vi "Message Handling Loop - UI.vi"(8 "error in":errorcluster, 9 "Message Queues in":T1, 10 "User Event Bundle":T2) -> (0 "error out":errorcluster)   [LabVIEW 2018]
uses:
  Type Defs/User Events.ctl
  Support/Message Queue/All Message Queues.ctl
  Support/Message Queue/Message Cluster.ctl
  Type Defs/UI Loop Data.ctl
  Type Defs/SR Cluster.ctl
  Type Defs/SR Status.ctl
  Type Defs/Filter Cluster.ctl
  Type Defs/Sorting Methods.ctl
  Support/Message Queue/Enqueue Message (Single).vi
  <vilib>/Utility/error.llb/Error Cluster From Error Code.vi
  <vilib>/ErrorRing/Error Ring.xnode
  Support/Message Queue/Message Queue.lvlib
  Support/User Events/User Events.lvlib
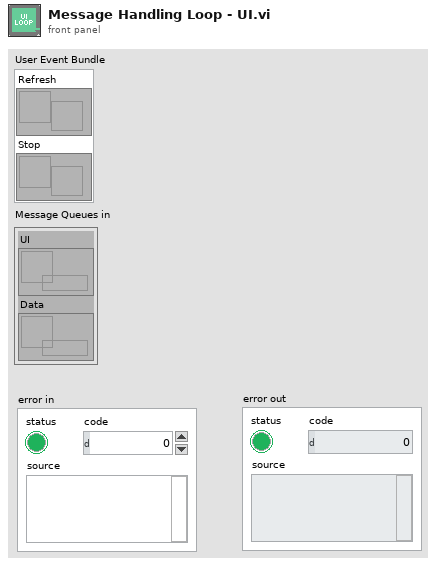
[diagram p1: front panel]
types:
  T1 = typedef "Message Queue.lvlib/All Message Queues.ctl" = cluster{"UI":refnum<queue>, "Data":refnum<queue>}
  T2 = typedef "User Events.ctl" = cluster{"Refresh":refnum<user-event>, "Stop":refnum<user-event>}
  T3 = typedef "UI Loop Data.ctl" = cluster{"SR Display List":T4[], "Filter Cluster":T6, "Exit":refnum<vi>, "Main VI":refnum<vi>, "Sorting":T7, "SR Display List":refnum<vi>, "Message":refnum<vi>, "UI":refnum<queue>, "Data":refnum<queue>}
  T4 = typedef "SR Cluster.ctl" = cluster{"Color":u32, "SR Number":i32, "SR Status":T5, "Name":string, "Summary":string, "Last Updated":timestamp, "SR Type":string, "Service Level":string, "Days Open":dbl, "Creation Date":timestamp}
  T5 = typedef "SR Status.ctl" = enum16{"Caller Abandoned", "Created in Error", "Expired", "Forum Resolved AE", "Forum Resolved Customer", "IN WORK", "IN WORK Collab with AES", "IN WORK Collab with PSE", "IN WORK Collab with SE", "IN WORK Customer Added Note", "IN WORK Escalation", "IN WORK Wait on Customer", "Open", "Potentially Resolved", "Presumed Resolved", "RMA Approved for Return", "Resolved", "Passed Off"}
  T6 = typedef "Filter Cluster.ctl" = cluster{"Show Resolved":bool, "Show Potentially Resolved":bool, "Show Passoffs":bool, "Show In Collab":bool}
  T7 = typedef "Sorting Methods.ctl" = enum16{"SR Status", "Most Recent", "SR Type", "SR Number"}
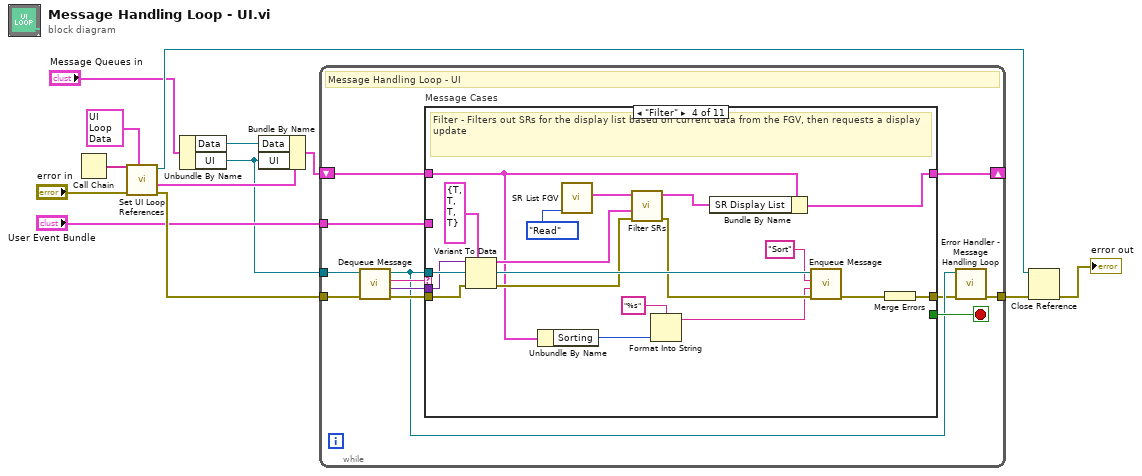
[diagram p0: block diagram]
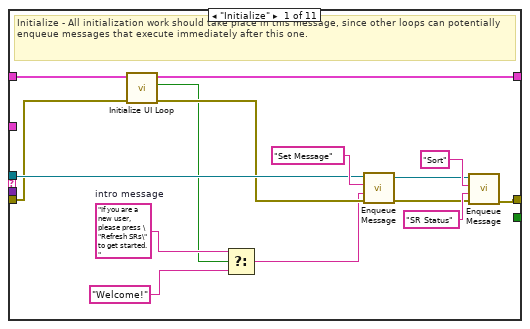
[diagram p2: hidden frame]
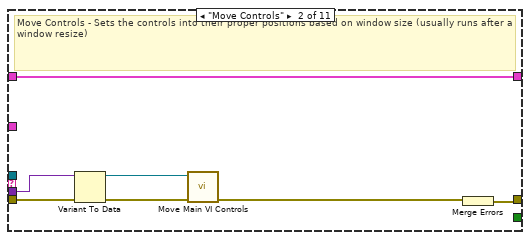
[diagram p3: hidden frame]
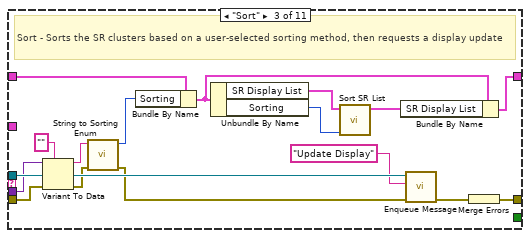
[diagram p4: hidden frame]
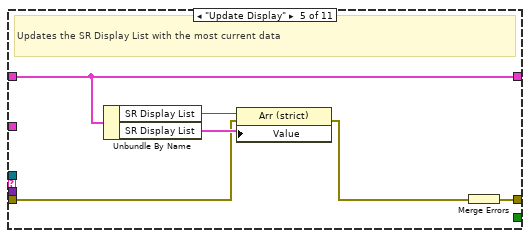
[diagram p5: hidden frame]
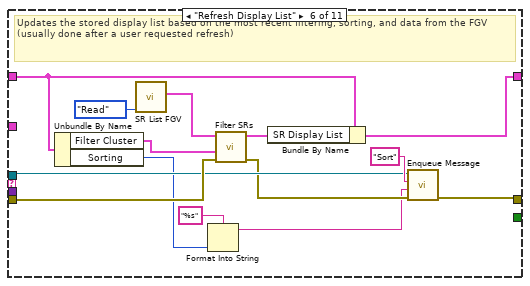
[diagram p6: hidden frame]
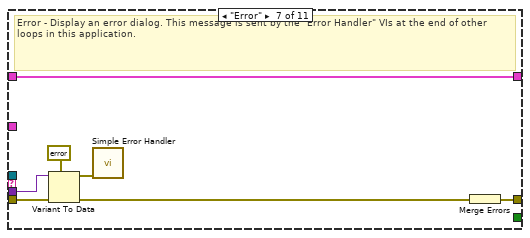
[diagram p7: hidden frame]
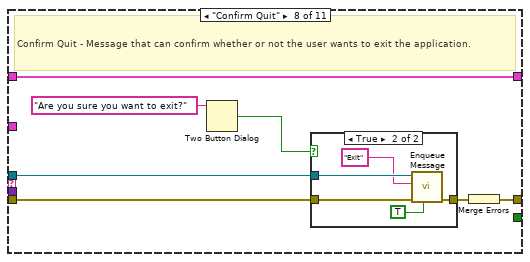
[diagram p8: hidden frame]
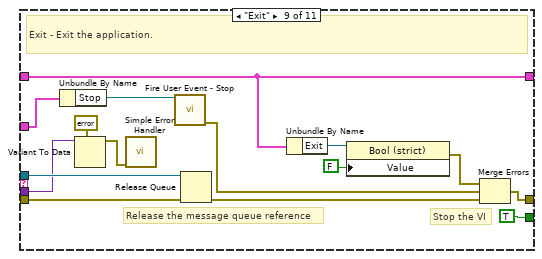
[diagram p10: hidden frame]
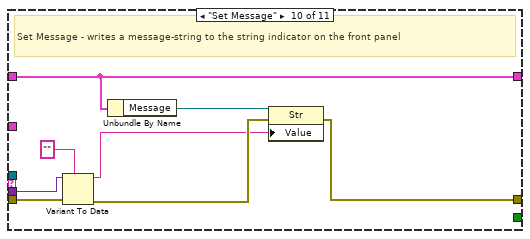
[diagram p11: hidden frame]
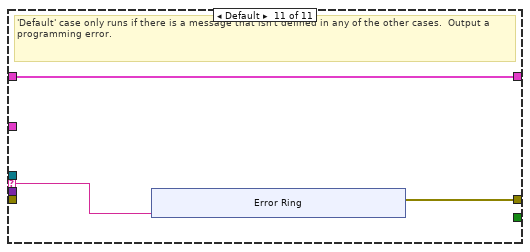
[diagram p12: hidden frame]
diagram:
  n1 = Call Chain() -> (call chain=w9:string[])
  n2 = call "Set UI Loop References.vi"("UI Data in"=T3 {"SR Display List"=[], "Filter Cluster"={"Show Resolved"=TRUE, "Show Potentially Resolved"=TRUE, "Show Passoffs"=TRUE, "Show In Collab"=TRUE}, "Exit"=refnum, "Main VI"=refnum, "Sorting"=enum."SR Status", "SR Display List"=refnum, "Message"=refnum, "UI"=refnum, "Data"=refnum}, "error in (no error)"="error in", "call chain"=w9) -> ("error out"=w13:errorcluster, "UI Data out"=w4:T3, "VI reference out"=w12:refnum<vi>)  [unwired: 6 in]
  n3 = Unbundle By Name("Message Queues in") -> ("Data"=w5:refnum<queue>, "UI"=w3:refnum<queue>)
  n4 = Bundle By Name(cluster=w4, "Data"=w5, "UI"=w3) -> (w1:T3)
  n5 = while {
    tunnel: w3 -> [w18]
    shift-right: [w24] -> _
    shift-left: w1 -> [w25]
    tunnel: w13 -> [w22]
    tunnel: [w16] -> w10
    tunnel: "User Event Bundle" -> [w14]
    stop <- w23 stop-if-true
    # "Message Handling Loop - UI"
    n6 = call "Dequeue Message.vi"("error in (no error)"=w22, "Message Queue"=w18) -> ("error out"=w21:errorcluster, "Message Data"=w19:variant, "Message"=w20:string, "dup Message Queue"=w17:refnum<queue>)  [unwired: 6 in]
    n7 = case "Message Cases" shown="\"Filter\"" w20 {
      selector: w20 -> [_ _ _ _ _ _ _ _ _ _ w146]
      tunnel: w17 -> [w34 _ w62 w80 _ w96 _ w112 w137 _ _]
      tunnel: w21 -> [w33 w46 w57 w71 w84 w98 w109 w116 w134 w143 _]
      tunnel: [w40 w42 w64 w82 w88 w94 w103 w114 w127 w139 w147] -> w15
      tunnel: w25 -> [w38 w47 w50 w68 w87 w93 w108 w115 w130 w145 w148]
      tunnel: [w39 w47 w59 w74 w87 w99 w108 w115 w130 w145 w148] -> w24
      tunnel: [_ _ _ _ _ _ _ _ TRUE _ _] -> w23
      tunnel: w19 -> [_ w44 w58 w72 _ _ w107 _ w131 w142 _]
      tunnel: w14 -> [_ _ _ _ _ _ _ _ w125 _ _]
      frame "Initialize" {
        w29 = "If you are a new user, please press \"Refresh SRs\" to get started."  # intro message
        # "Initialize - All initialization work should take place in this message, since other loops can potentially enqueue messages that execute immediately after this one."
        n8 = call "Initialize UI Loop.vi"("error in"=w33, "UI Data in"=w38) -> ("error out"=w32:errorcluster, "new user?"=w26:bool, "UI Data out 2"=w39:T3)  [unwired: 7 in]
        n9 = Select(t=w29, s=w26, f="Welcome!") -> (s? t:f=w27:string)
        n10 = call-poly "Enqueue Message.vi"("error in (no error)"=w32, "Message Data"=w27, "Message"="Set Message", "Message Queue"=w34) -> ("error out"=w31:errorcluster, "dup Message Queue"=w30:refnum<queue>)  [unwired: 6 in]
        n11 = call-poly "Enqueue Message.vi"("error in (no error)"=w31, "Message Data"="SR Status" ("Message"), "Message"="Sort", "Message Queue"=w30) -> ("error out"=w40:errorcluster)  [unwired: 6 in, 1 out]
      }
      frame "Move Controls" {
        # "Move Controls - Sets the controls into their proper positions based on window size (usually runs after a window resize)"
        n12 = Variant To Data(error in=w46, Variant=w44) -> (data=w45:refnum<vi>, error out=w43:errorcluster)  [unwired: 1 in]
        n13 = call "Move Main VI Controls.vi"("error in"=w43, "VIRef in"=w45) -> ("error out"=w41:errorcluster)  [unwired: 9 in]
        n14 = Merge Errors(w41) -> (w42:errorcluster)
      }
      frame "Sort" {
        # "Sort - Sorts the SR clusters based on a user-selected sorting method, then requests a display update"
        n15 = Variant To Data(error in=w57, type="", Variant=w58) -> (data=w56:string, error out=w54:errorcluster)
        n16 = call "String to Sorting Enum.vi"("error in"=w54, "string in"=w56) -> ("error out"=w53:errorcluster, "Sorting"=w49:T7)  [unwired: 8 in]
        n17 = Bundle By Name(cluster=w50, "Sorting"=w49) -> (w48:T3)
        n18 = Unbundle By Name(w48) -> ("SR Display List"=w60:T4[], "Sorting"=w51:T7)
        n19 = call "Sort SR List.vi"("Sorting"=w51, "list in"=w60) -> ("list out"=w52:T4[])  [unwired: 9 in]
        n20 = Bundle By Name(cluster=w48, "SR Display List"=w52) -> (w59:T3)
        n21 = call-poly "Enqueue Message.vi"("error in (no error)"=w53, "Message"="Update Display", "Message Queue"=w62) -> ("error out"=w63:errorcluster)  [unwired: 7 in, 1 out]
        n22 = Merge Errors(w63) -> (w64:errorcluster)
      }
      frame "Filter" {
        # "Filter - Filters out SRs for the display list based on current data from the FGV, then requests a display update"
        n23 = Variant To Data(error in=w71, type=T6 {"Show Resolved"=TRUE, "Show Potentially Resolved"=TRUE, "Show Passoffs"=TRUE, "Show In Collab"=TRUE} ("Filter Cluster"), Variant=w72) -> (data=w69:T6, error out=w70:errorcluster)
        n24 = Unbundle By Name(w68) -> ("Sorting"=w66:T7)
        n25 = call "SR List FGV.vi"("Operation"=enum16{"Initialize", "Write", "Read", "Clear"}."Read") -> ("list out"=w77:T4[])  [unwired: 9 in, 1 out]
        n26 = call "Filter SRs.vi"("error in"=w70, "Filter Cluster"=w69, "list in"=w77) -> ("error out"=w78:errorcluster, "list out"=w75:T4[])  [unwired: 7 in]
        n27 = Format Into String(format string="%s", w66) -> (resulting string=w65:string)  [unwired: 2 in, 1 out]
        n28 = Bundle By Name(cluster=w68, "SR Display List"=w75) -> (w74:T3)
        n29 = call-poly "Enqueue Message.vi"("error in (no error)"=w78, "Message Data"=w65, "Message"="Sort", "Message Queue"=w80) -> ("error out"=w81:errorcluster)  [unwired: 6 in, 1 out]
        n30 = Merge Errors(w81) -> (w82:errorcluster)
      }
      frame "Update Display" {
        # "Updates the SR Display List with the most current data"
        n31 = Unbundle By Name(w87) -> ("SR Display List"=w86:refnum<vi>, "SR Display List"=w85:T4[])
        n32 = property class="Arr (strict)"(reference=w86, error in=w84, "Value"=w85) -> (error out=w83:errorcluster)  [unwired: 1 out]
        n33 = Merge Errors(w83) -> (w88:errorcluster)
      }
      frame "Refresh Display List" {
        # "Updates the stored display list based on the most recent filtering, sorting, and data from the FGV (usually done after a user requested refresh)"
        n34 = Unbundle By Name(w93) -> ("Filter Cluster"=w90:T6, "Sorting"=w89:T7)
        n35 = call "SR List FGV.vi"("Operation"=enum16{"Initialize", "Write", "Read", "Clear"}."Read") -> ("list out"=w101:T4[])  [unwired: 9 in, 1 out]
        n36 = Format Into String(format string="%s", w89) -> (resulting string=w91:string)  [unwired: 2 in, 1 out]
        n37 = call "Filter SRs.vi"("error in"=w98, "Filter Cluster"=w90, "list in"=w101) -> ("error out"=w95:errorcluster, "list out"=w100:T4[])  [unwired: 7 in]
        n38 = Bundle By Name(cluster=w93, "SR Display List"=w100) -> (w99:T3)
        n39 = call-poly "Enqueue Message.vi"("error in (no error)"=w95, "Message Data"=w91, "Message"="Sort", "Message Queue"=w96) -> ("error out"=w94:errorcluster)  [unwired: 6 in, 1 out]
      }
      frame "Error" {
        # "Error - Display an error dialog. This message is sent by the \"Error Handler\" VIs at the end of other loops in this application."
        n40 = Variant To Data(error in=w109, type=errorcluster {"status"=FALSE, "code"=0, "source"=""} ("error constant"), Variant=w107) -> (data=w105:errorcluster, error out=w104:errorcluster)
        n41 = call <vilib>:"Simple Error Handler.vi"("error in (no error)"=w105) -> ()  [unwired: 4 in, 5 out]
        n42 = Merge Errors(w104) -> (w103:errorcluster)
      }
      frame "Confirm Quit" {
        # "Confirm Quit - Message that can confirm whether or not the user wants to exit the application."
        n43 = Two Button Dialog(message="Are you sure you want to exit?") -> (T button?=w110:bool)  [unwired: 2 in]
        n44 = case shown="True" w110 {
          tunnel: w116 -> [w117 w122]
          tunnel: [w117 w121] -> w113
          tunnel: w112 -> [_ w120]
          frame False {
          }
          frame True {
            n45 = call-poly "Enqueue Message.vi"("Priority Message? (F)"=TRUE, "error in (no error)"=w122, "Message"="Exit", "Message Queue"=w120) -> ("error out"=w121:errorcluster)  [unwired: 6 in, 1 out]
          }
        }
        n46 = Merge Errors(w113) -> (w114:errorcluster)
      }
      frame "Exit" {
        # "Stop the VI"
        # "Release the message queue reference"
        # "Exit - Exit the application."
        n47 = Unbundle By Name(w125) -> ("Stop"=w124:refnum<user-event>)
        n48 = Variant To Data(type=errorcluster {"status"=FALSE, "code"=0, "source"=""} ("error constant"), Variant=w131) -> (data=w132:errorcluster)  [unwired: 1 in, 1 out]
        n49 = call <vilib>:"Simple Error Handler.vi"("error in (no error)"=w132) -> ()  [unwired: 4 in, 5 out]
        n50 = call "Fire User Event - Stop.vi"("Stop"=w124) -> ("error out"=w123:errorcluster)  [unwired: 10 in]
        n51 = Release Queue(queue=w137, error in (no error)=w134) -> (error out=w135:errorcluster)  [unwired: 1 in, 2 out]
        n52 = Unbundle By Name(w130) -> ("Exit"=w126:refnum<vi>)
        n53 = property class="Bool (strict)"(reference=w126, "Value"=FALSE) -> (error out=w128:errorcluster)  [unwired: 1 in, 1 out]
        n54 = Merge Errors(w128, w123, w135) -> (w127:errorcluster)
      }
      frame "Set Message" {
        # "Set Message - writes a message-string to the string indicator on the front panel"
        n55 = Variant To Data(error in=w143, type="", Variant=w142) -> (data=w138:string, error out=w140:errorcluster)
        n56 = Unbundle By Name(w145) -> ("Message"=w144:refnum<vi>)
        n57 = property class="Str"(reference=w144, error in=w140, "Value"=w138) -> (error out=w139:errorcluster)  [unwired: 1 out]
      }
      frame Default {
        # "'Default' case only runs if there is a message that isn't defined in any of the other cases.  Output a programming error."
        n58 = xnode "Error Ring"("parameter 0"=w146) -> ("error out"=w147:errorcluster)
      }
    }
    n59 = call "Error Handler - Message Handling Loop.vi"("error in (no error)"=w15, "Message Queue"=w17) -> ("dup error in"=w16:errorcluster)  [unwired: 8 in, 1 out]
  }
  n60 = Close Reference(reference=w12, error in (no error)=w10) -> (error out=→"error out":errorcluster)
